vi "DownloadDataNewWindow.vi"() -> (0 "Data aquired?":bool, 1 "Yaxis":dbl[](array[numeric]), 2 "Xaxis":dbl[](array[numeric]), 3 "name (change?)":string, 6 "Single FIle?":bool, 7 "Multiple Data":cluster{dbl[], dbl[]}[](array[cluster]))   [LabVIEW 2020]
uses:
  TypeDefDownloadData.ctl
panel:
  in  "Abort":bool
  in  "Ready":bool
  in  "Tab Control":T1(tab)
  in  "Remove negative values":bool
  in  "Delete point":bool
  in  "Choose value (X)":dbl
  in  "Find Data":bool
  in  "DownloadMenu":u16(ring) items=["Headless", "With Header"]
  in  "Divide (Integration time)":dbl
  in  "Multiply?":bool
  out "Data":cluster{dbl[], dbl[]}(graph)
  in  "Name (change?)":string
  in  "Update data":bool
  in  "Replace":string
  in  "Search":string
  in  "Downloaded data from file":string
  in  "Use this data":bool
  in  "Separator":u16(ring) items=["Current separator", "Tab", "Space", "Blank"]
  in  "Find Data MultiFolder":bool
  out "DataMultiFolder":cluster{dbl[], dbl[]}[](graph)
  in  "path":path
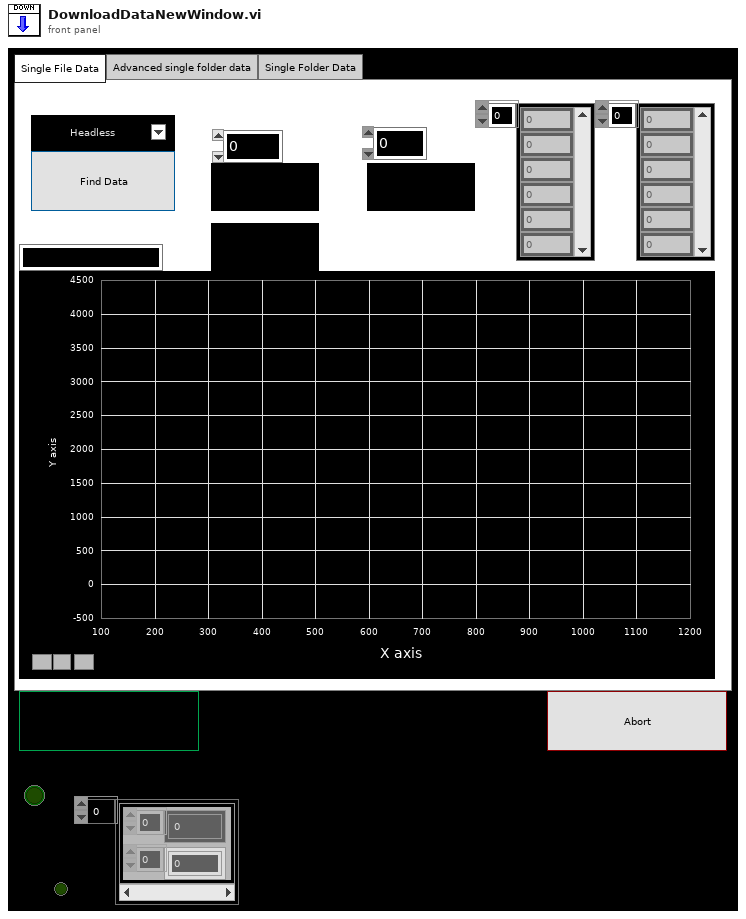
[diagram p1: front panel]
types:
  T1 = enum32{"Single File Data", "Advanced single folder data", "Single Folder Data"}
  T2 = typedef "TypeDefDownloadData.ctl" = enum16{"Wait", "DownloadData", "Multiply", "Exit", "Abort", "Folder", "Point", "UseString", "UpdateString", "AbsVal"}
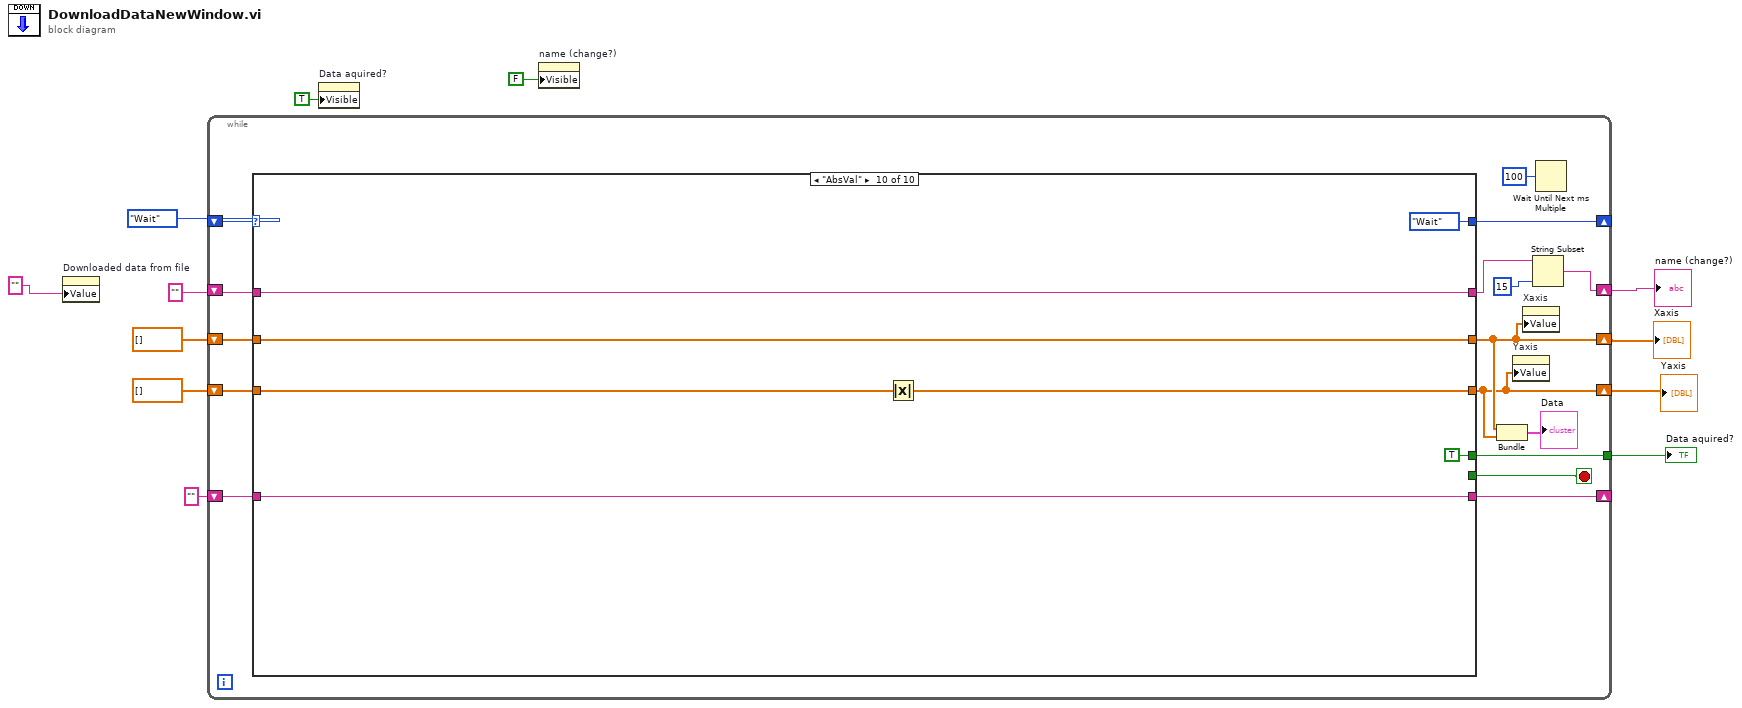
[diagram p0: block diagram]
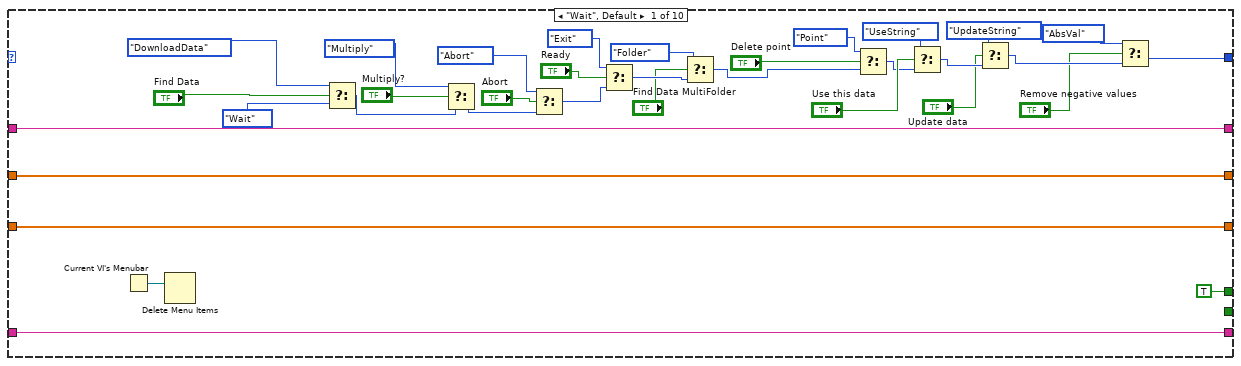
[diagram p2: hidden frame]
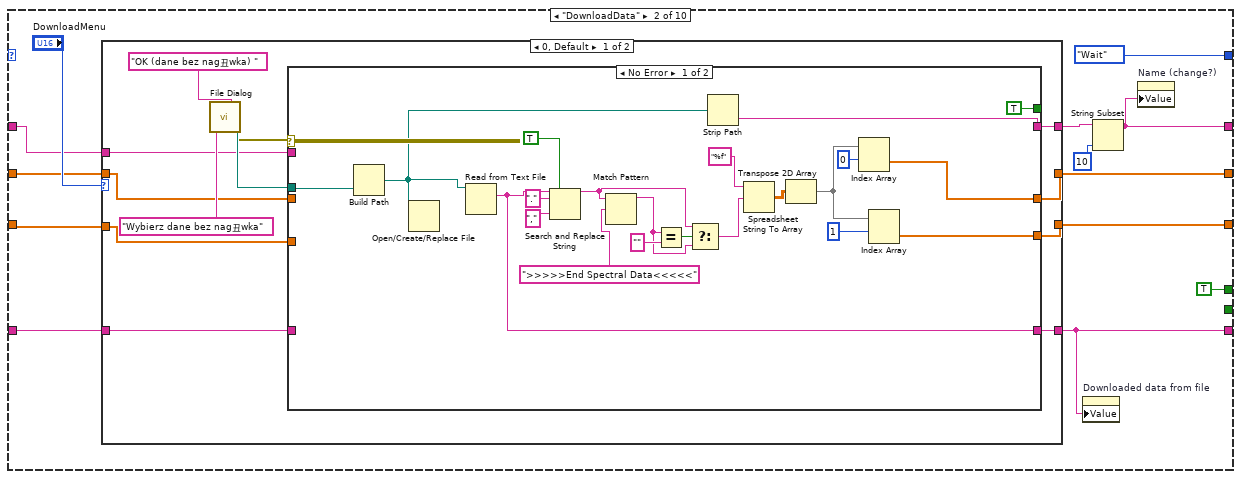
[diagram p3: hidden frame]
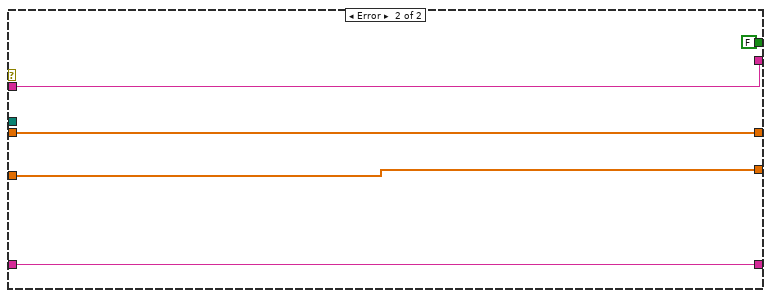
[diagram p4: hidden frame]
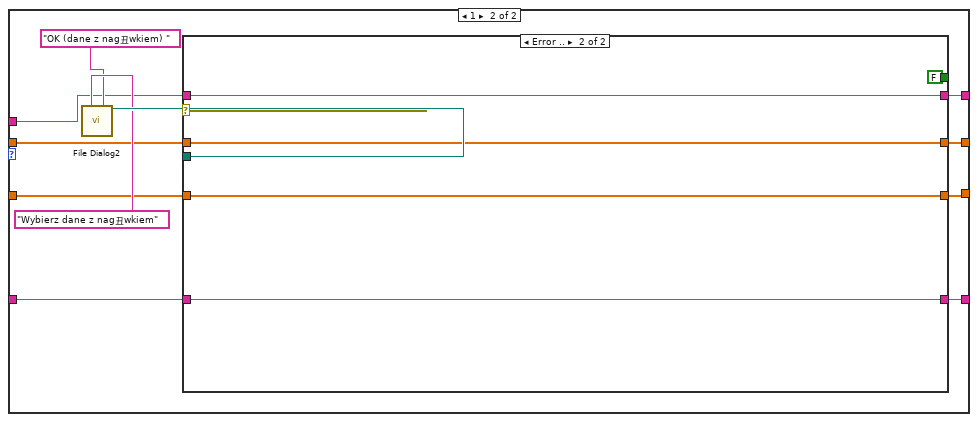
[diagram p5: hidden frame]
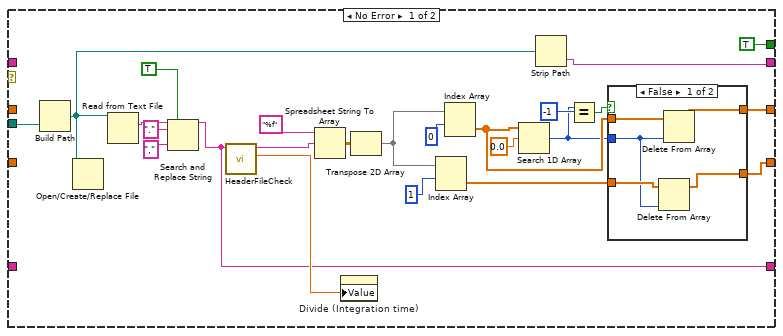
[diagram p6: hidden frame]
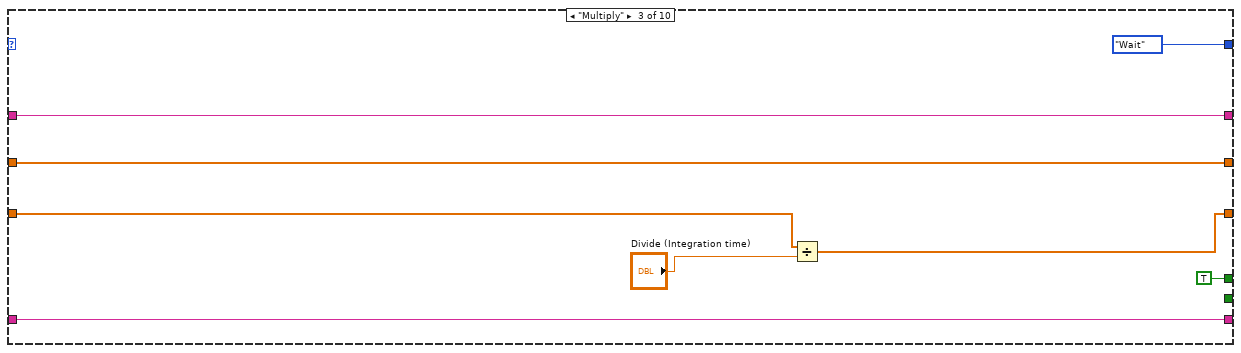
[diagram p8: hidden frame]
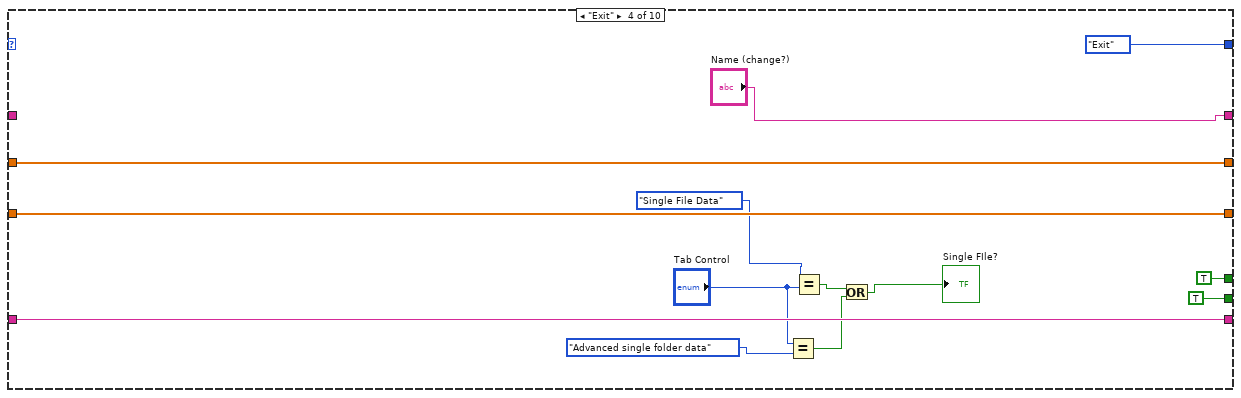
[diagram p9: hidden frame]
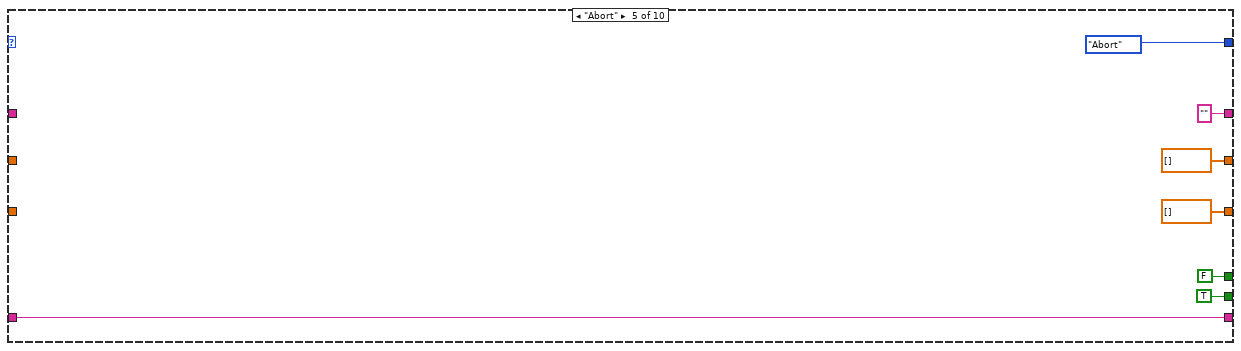
[diagram p10: hidden frame]
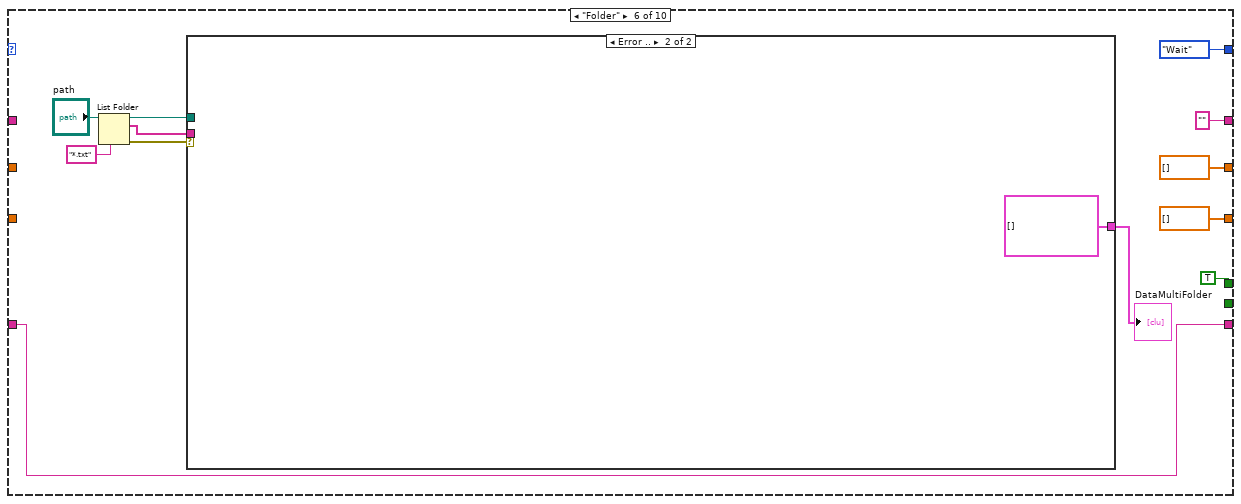
[diagram p11: hidden frame]
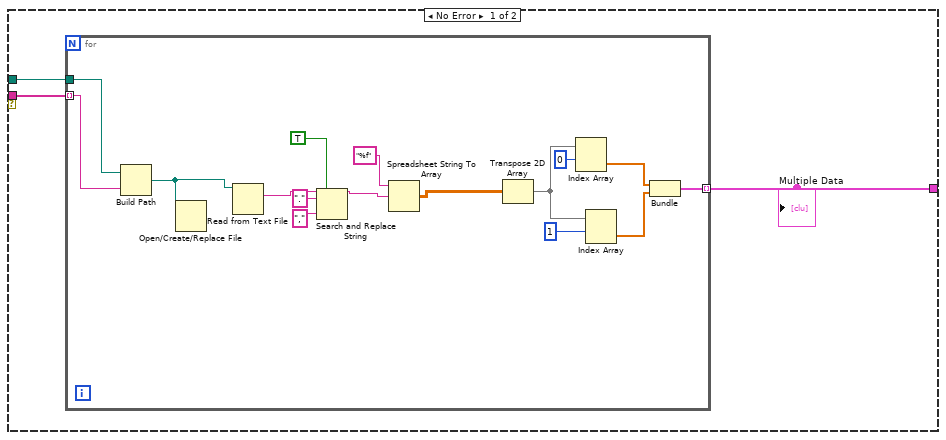
[diagram p12: hidden frame]
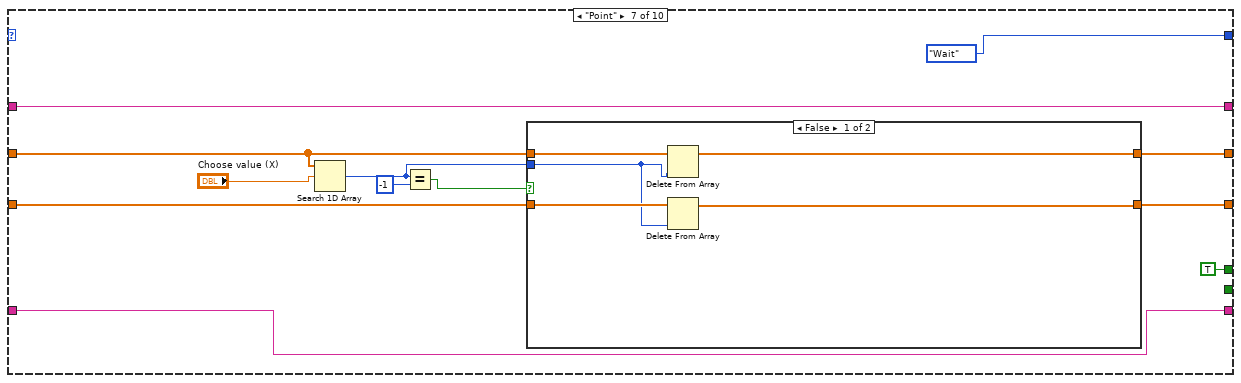
[diagram p13: hidden frame]
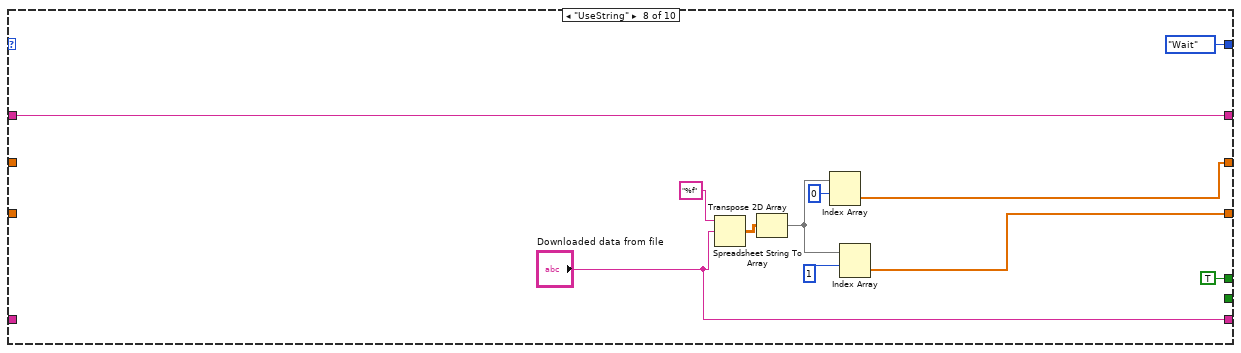
[diagram p15: hidden frame]
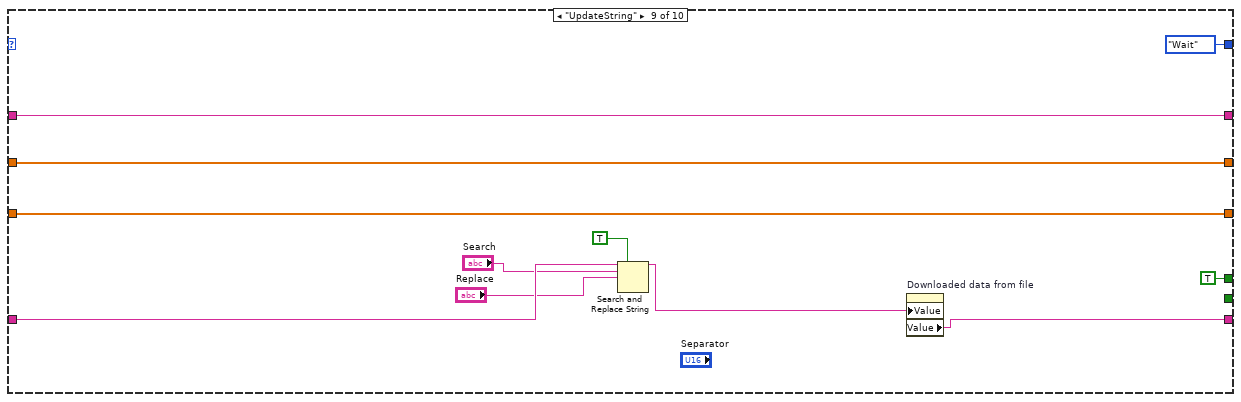
[diagram p16: hidden frame]
diagram:
  n1 = property on="Downloaded data from file" class="Str"("Value"="" ("result string")) -> ()  [unwired: 2 in, 2 out]
  n2 = while {
    shift-right: [w20] -> w6
    shift-left: dbl[] [] -> [w24]
    shift-right: [w19] -> w11
    shift-left: dbl[] [] -> [w23]
    shift-right: [w15] -> w12
    shift-left: "" ("name") -> [w25]
    shift-right: [w27] -> _
    shift-left: TypeDefDownloadData."Wait" -> [w26]
    tunnel: [w22] -> w5
    shift-right: [w14] -> _
    shift-left: "" ("result string") -> [w13]
    stop <- w21 stop-if-true
    n3 = case shown="\"AbsVal\"" w26 {
      tunnel: [w61 w69 w169 "Name (change?)" "" ("name") "" ("name") w233 w251 w260 w268] -> w16
      tunnel: [w47 w72 w168 w181 dbl[] [] dbl[] [] w227 w243 w259 w267] -> w20
      tunnel: [w46 w71 w165 w180 dbl[] [] dbl[] [] w230 w242 w258 w263] -> w19
      tunnel: [w31 TypeDefDownloadData."Wait" TypeDefDownloadData."Wait" TypeDefDownloadData."Exit" TypeDefDownloadData."Abort" TypeDefDownloadData."Wait" TypeDefDownloadData."Wait" TypeDefDownloadData."Wait" TypeDefDownloadData."Wait" TypeDefDownloadData."Wait"] -> w27
      tunnel: w25 -> [w61 w65 w169 _ _ _ w233 w251 w260 w268]
      tunnel: w24 -> [w47 w67 w168 w181 _ _ w228 _ w259 w267]
      tunnel: w23 -> [w46 w66 w166 w180 _ _ w229 _ w258 w264]
      tunnel: [_ _ _ TRUE TRUE _ _ _ _ _] -> w21
      tunnel: [TRUE TRUE TRUE TRUE FALSE TRUE TRUE TRUE TRUE TRUE] -> w22
      tunnel: [w33 w63 w162 w176 w183 w190 w223 "Downloaded data from file" w252 w266] -> w14
      tunnel: w13 -> [w33 w64 w162 w176 w183 w190 w223 _ w257 w266]
      frame "Wait", Default {
        n4 = Current VI's Menubar() -> (w53:refnum<k9>)
        n5 = Delete Menu Items(9:w53) -> ()  [unwired: 3 in, 2 out]
        n6 = Select(t=TypeDefDownloadData."DownloadData", s="Find Data", f=TypeDefDownloadData."Wait") -> (s? t:f=w60:T2)
        n7 = Select(t=TypeDefDownloadData."Multiply", s="Multiply?", f=w60) -> (s? t:f=w58:T2)
        n8 = Select(t=TypeDefDownloadData."Abort", s="Abort", f=w58) -> (s? t:f=w50:T2)
        n9 = Select(t=TypeDefDownloadData."Exit", s="Ready", f=w50) -> (s? t:f=w45:T2)
        n10 = Select(t=TypeDefDownloadData."Folder", s="Find Data MultiFolder", f=w45) -> (s? t:f=w41:T2)
        n11 = Select(t=TypeDefDownloadData."Point", s="Delete point", f=w41) -> (s? t:f=w38:T2)
        n12 = Select(t=TypeDefDownloadData."UseString", s="Use this data", f=w38) -> (s? t:f=w36:T2)
        n13 = Select(t=TypeDefDownloadData."UpdateString", s="Update data", f=w36) -> (s? t:f=w32:T2)
        n14 = Select(t=TypeDefDownloadData."AbsVal", s="Remove negative values", f=w32) -> (s? t:f=w31:T2)
      }
      frame "DownloadData" {
        n15 = case shown="0, Default" "DownloadMenu" {
          tunnel: [w83 w121] -> w70
          tunnel: [w82 w120] -> w72
          tunnel: [w81 w119] -> w71
          tunnel: w67 -> [w80 w118]
          tunnel: w66 -> [w79 w117]
          tunnel: w65 -> [w78 w116]
          tunnel: [w77 w115] -> w63
          tunnel: w64 -> [w76 w114]
          frame 0, Default {
            n16 = call "File Dialog"("prompt"="Wybierz dane bez nag丑wka" ("button label"), "button label"="OK (dane bez nag丑wka) ") -> ("selected path"=w87:path, "error out"=w86:errorcluster)  [unwired: 10 in, 2 out]
            n17 = case shown="No Error" w86 {
              tunnel: w87 -> [w108 _]
              tunnel: [w104 w110] -> w83
              tunnel: [TRUE ("Czy dane pobrane?") FALSE ("Czy dane pobrane?")] -> _
              tunnel: [w96 w112] -> w82
              tunnel: [w95 w111] -> w81
              tunnel: w80 -> [_ w112]
              tunnel: w79 -> [_ w111]
              tunnel: w78 -> [_ w110]
              tunnel: [w88 w109] -> w77
              tunnel: w76 -> [_ w109]
              frame No Error {
                n18 = Build Path(name or relative path=w108) -> (appended path=w97:path)  [unwired: 1 in]
                n19 = Open/Create/Replace File(file path (use dialog)=w97) -> ()  [unwired: 5 in, 3 out]
                n20 = Read from Text File(file (use dialog)=w97) -> (text=w88:string)  [unwired: 3 in, 3 out]
                n21 = Search and Replace String(replace all?=TRUE ("replace all? (F)"), input string=w88, search string=".", replace string="," ("replace string (\"\")")) -> (result string=w90:string)  [unwired: 4 in, 3 out]
                n22 = Match Pattern(string=w90, regular expression=">>>>>End Spectral Data<<<<<") -> (before substring=w91:string)  [unwired: 1 in, 3 out]
                n23 = Equal?(x=w91, y="") -> (x = y?=w94:bool)
                n24 = Select(t=w90, s=w94, f=w91) -> (s? t:f=w89:string)
                n25 = Strip Path(path=w97) -> (name=w104:string)  [unwired: 1 out]
                n26 = Spreadsheet String To Array(format string="%f", spreadsheet string=w89) -> (array=w98:dbl[][])  [unwired: 2 in]
                n27 = Transpose 2D Array(2D array=w98) -> (transposed array=w105:dbl[][])
                n28 = Index Array(array=w105, index (row)=0) -> (element=w96:dbl[])  [unwired: 1 in]
                n29 = Index Array(array=w105, index (row)=1) -> (element=w95:dbl[])  [unwired: 1 in]
              }
              frame Error {
              }
            }
          }
          frame 1 {
            n30 = call "File Dialog2"("prompt"="Wybierz dane z nag丑wkiem" ("button label"), "button label"="OK (dane z nag丑wkiem) ") -> ("selected path"=w125:path, "error out"=w124:errorcluster)  [unwired: 10 in, 2 out]
            n31 = case shown="Error .." w124 {
              tunnel: w125 -> [w149 _]
              tunnel: [w128 w158] -> w121
              tunnel: [TRUE ("Czy dane pobrane?") FALSE ("Czy dane pobrane?")] -> _
              tunnel: [w130 w160] -> w120
              tunnel: [w133 w159] -> w119
              tunnel: w118 -> [_ w160]
              tunnel: w117 -> [_ w159]
              tunnel: w116 -> [_ w158]
              tunnel: [w126 w157] -> w115
              tunnel: w114 -> [_ w157]
              frame No Error {
                n32 = Build Path(name or relative path=w149) -> (appended path=w139:path)  [unwired: 1 in]
                n33 = Open/Create/Replace File(file path (use dialog)=w139) -> ()  [unwired: 5 in, 3 out]
                n34 = Read from Text File(file (use dialog)=w139) -> (text=w127:string)  [unwired: 3 in, 3 out]
                n35 = Search and Replace String(replace all?=TRUE ("replace all? (F)"), input string=w127, search string=".", replace string="," ("replace string (\"\")")) -> (result string=w126:string)  [unwired: 4 in, 3 out]
                n36 = call "HeaderFileCheck.vi"("result string in"=w126) -> ("Integration time"=w138:dbl, "result string out"=w137:string)  [unwired: 9 in]
                n37 = Spreadsheet String To Array(format string="%f", spreadsheet string=w137) -> (array=w140:dbl[][])  [unwired: 2 in]
                n38 = property on="Divide (Integration time)" class="DigNum (strict)"("Value"=w138) -> ()  [unwired: 2 in, 2 out]
                n39 = Transpose 2D Array(2D array=w140) -> (transposed array=w146:dbl[][])
                n40 = Index Array(array=w146, index (row)=1) -> (element=w132:dbl[])  [unwired: 1 in]
                n41 = Index Array(array=w146, index (row)=0) -> (element=w131:dbl[])  [unwired: 1 in]
                n42 = Search 1D Array(1D array=w131, element=0.0) -> (index of element=w129:i32)  [unwired: 1 in]
                n43 = Strip Path(path=w139) -> (name=w128:string)  [unwired: 1 out]
                n44 = Equal?(x=w129, y=-1) -> (x = y?=w134:bool)
                n45 = case shown="False" w134 {
                  tunnel: [w152 w156] -> w133
                  tunnel: w132 -> [w153 w156]
                  tunnel: w131 -> [w154 w155]
                  tunnel: [w151 w155] -> w130
                  tunnel: w129 -> [w150 _]
                  frame False {
                    n46 = Delete From Array(array=w153, index=w150) -> (array with subset deleted=w152:dbl[])  [unwired: 1 in, 1 out]
                    n47 = Delete From Array(array=w154, index=w150) -> (array with subset deleted=w151:dbl[])  [unwired: 1 in, 1 out]
                  }
                  frame True {
                  }
                }
              }
              frame Error {
              }
            }
          }
        }
        n48 = property on="Downloaded data from file" class="Str"("Value"=w63) -> ()  [unwired: 2 in, 2 out]
        n49 = String Subset(string=w70, length (rest)=10 ("length (rest)")) -> (substring=w69:string)  [unwired: 1 in]
        n50 = property on="Name (change?)" class="Str"("Value"=w69) -> ()  [unwired: 2 in, 2 out]
      }
      frame "Multiply" {
        n51 = Divide(x=w166, y="Divide (Integration time)") -> (x/y=w165:dbl[])
      }
      frame "Exit" {
        n52 = Equal?(x="Tab Control", y=T1."Advanced single folder data" ("Tab Control")) -> (x = y?=w171:bool)
        n53 = Equal?(x=T1."Single File Data" ("Tab Control"), y="Tab Control") -> (x = y?=w175:bool)
        n54 = Or(x=w175, y=w171) -> (x .or. y?=→"Single FIle?":bool)
      }
      frame "Abort" {
      }
      frame "Folder" {
        n55 = List Folder(path="path", pattern="*.txt") -> (path out=w196:path, filenames=w192:string[], error out=w197:errorcluster)  [unwired: 2 in, 1 out]
        n56 = case shown="Error .." w197 {
          tunnel: w192 -> [w204 _]
          tunnel: w196 -> [w203 _]
          tunnel: [w202 cluster{dbl[], dbl[]}[] []] -> w195
          frame No Error {
            n57 = for {
              tunnel: w204 -> [w209] mode=indexing
              tunnel: w203 -> [w208]
              tunnel: [w205] -> w202 mode=indexing
              n58 = Build Path(base path=w208, name or relative path=w209) -> (appended path=w210:path)
              n59 = Open/Create/Replace File(file path (use dialog)=w210) -> ()  [unwired: 5 in, 3 out]
              n60 = Read from Text File(file (use dialog)=w210) -> (text=w216:string)  [unwired: 3 in, 3 out]
              n61 = Search and Replace String(replace all?=TRUE ("replace all? (F)"), input string=w216, search string=".", replace string="," ("replace string (\"\")")) -> (result string=w212:string)  [unwired: 4 in, 3 out]
              n62 = Spreadsheet String To Array(format string="%f", spreadsheet string=w212) -> (array=w211:dbl[][])  [unwired: 2 in]
              n63 = Transpose 2D Array(2D array=w211) -> (transposed array=w218:dbl[][])
              n64 = Index Array(array=w218, index (row)=0) -> (element=w207:dbl[])  [unwired: 1 in]
              n65 = Index Array(array=w218, index (row)=1) -> (element=w206:dbl[])  [unwired: 1 in]
              n66 = Bundle(w207, w206) -> (w205:cluster{dbl[], dbl[]})  [unwired: 1 in]
            }
            "Multiple Data" <- w202
          }
          frame Error {
          }
        }
        "DataMultiFolder" <- w195
      }
      frame "Point" {
        n67 = Search 1D Array(1D array=w228, element="Choose value (X)") -> (index of element=w224:i32)  [unwired: 1 in]
        n68 = Equal?(x=w224, y=-1) -> (x = y?=w225:bool)
        n69 = case shown="False" w225 {
          tunnel: [w235 w240] -> w230
          tunnel: w229 -> [w236 w240]
          tunnel: w228 -> [w238 w239]
          tunnel: [w237 w239] -> w227
          tunnel: w224 -> [w234 _]
          frame False {
            n70 = Delete From Array(array=w238, index=w234) -> (array with subset deleted=w237:dbl[])  [unwired: 1 in, 1 out]
            n71 = Delete From Array(array=w236, index=w234) -> (array with subset deleted=w235:dbl[])  [unwired: 1 in, 1 out]
          }
          frame True {
          }
        }
      }
      frame "UseString" {
        n72 = Spreadsheet String To Array(format string="%f", spreadsheet string="Downloaded data from file") -> (array=w244:dbl[][])  [unwired: 2 in]
        n73 = Transpose 2D Array(2D array=w244) -> (transposed array=w246:dbl[][])
        n74 = Index Array(array=w246, index (row)=0) -> (element=w243:dbl[])  [unwired: 1 in]
        n75 = Index Array(array=w246, index (row)=1) -> (element=w242:dbl[])  [unwired: 1 in]
      }
      frame "UpdateString" {
        n76 = Search and Replace String(replace all?=TRUE ("replace all? (F)"), input string=w257, search string="Search", replace string="Replace") -> (result string=w254:string)  [unwired: 4 in, 3 out]
        n77 = property on="Downloaded data from file" class="Str"("Value"=w254) -> ("Value"=w252:string)  [unwired: 2 in, 2 out]
      }
      frame "AbsVal" {
        n78 = Absolute Value(x=w264) -> (abs(x)=w263:dbl[])
      }
    }
    n79 = Bundle(w20, w19) -> (→"Data":cluster{dbl[], dbl[]})  [unwired: 1 in]
    n80 = property on="Yaxis" class="Arr (strict)"("Value"=w19) -> ()  [unwired: 2 in, 2 out]
    n81 = property on="Xaxis" class="Arr (strict)"("Value"=w20) -> ()  [unwired: 2 in, 2 out]
    n82 = String Subset(string=w16, length (rest)=15 ("length (rest)")) -> (substring=w15:string)  [unwired: 1 in]
    n83 = Wait Until Next ms Multiple(millisecond multiple=u32 100) -> ()  [unwired: 1 out]
  }
  "name (change?)" <- w12
  "Xaxis" <- w6
  "Yaxis" <- w11
  "Data aquired?" <- w5
  n84 = property on="Data aquired?" class="Bool (strict)"("Visible"=TRUE) -> ()  [unwired: 2 in, 2 out]
  n85 = property on="name (change?)" class="Str"("Visible"=FALSE) -> ()  [unwired: 2 in, 2 out]
